vi "aggregation-lifetime-management.vi"(8 "error in (no error)":errorcluster) -> (0 "error out":errorcluster)   [LabVIEW 2013]
uses:
  src/SMO/SMO.lvclass
  <vilib>/addons/_JKI Toolkits/Caraya/classes/Test/Test.lvclass
  <vilib>/addons/_JKI Toolkits/Caraya/classes/Assert/Assert.lvclass
panel:
  # "<< Error 1556 illustrates a bug with version 1.1.7.31 \n\n(Essentially because B is destroyed by top-level before A is stopped, and A depends on B that no longer exists on stopping... this error should be handled by framework. Reverse the launching order to demonstrate bug is lifetime-related)"
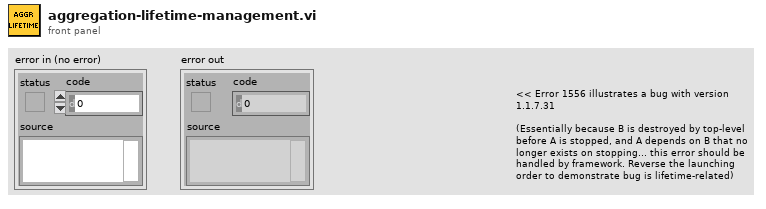
[diagram p1: front panel]
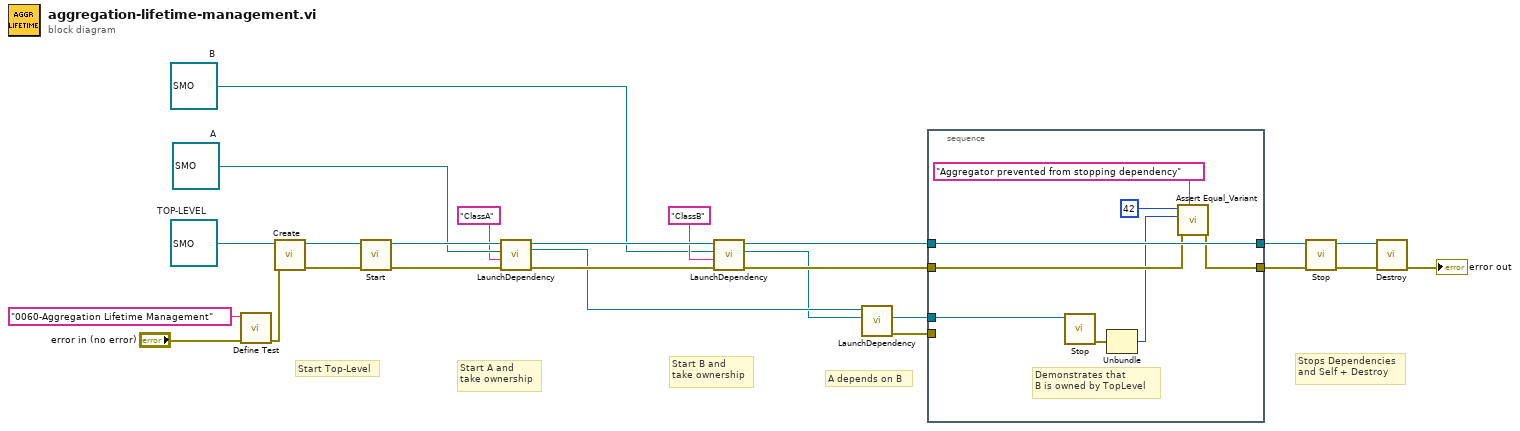
[diagram p0: block diagram]
diagram:
  w18 = refnum<class "SMO.lvclass"> refnum  # B
  w22 = refnum<class "SMO.lvclass"> refnum  # A
  w25 = refnum<class "SMO.lvclass"> refnum  # TOP-LEVEL
  # "Stops Dependencies\nand Self + Destroy"
  # "A depends on B"
  # "Start B and\ntake ownership"
  # "Start A and\ntake ownership"
  # "Start Top-Level"
  n1 = call <vilib>:"Define Test.vi"("error in (no error)"="error in (no error)", "Label (VI Title)"="0060-Aggregation Lifetime Management") -> ("error out"=w1:errorcluster)  [unwired: 9 in]
  n2 = call "Create.vi"("error in (no error)"=w1, "SMO"=w25) -> ("error out"=w16:errorcluster, "SMO out"=w24:refnum<class "SMO.lvclass">)  [unwired: 7 in, 1 out]
  n3 = call "Start.vi"("error in (no error)"=w16, "SMO"=w24) -> ("error out"=w17:errorcluster, "SMO out"=w23:refnum<class "SMO.lvclass">)  [unwired: 8 in]
  n4 = call "LaunchDependency.vi"("error in (no error)"=w17, "Dependency Name"="ClassA", "Dependency Type"=w22, "SMO in"=w23) -> ("error out"=w15:errorcluster, "Dependency Reference"=w6:refnum<class "SMO.lvclass">, "SMO out"=w20:refnum<class "SMO.lvclass">)  [unwired: 4 in, 1 out]
  n5 = call "LaunchDependency.vi"("error in (no error)"=w15, "Dependency Name"="ClassB", "Dependency Type"=w18, "SMO in"=w20) -> ("error out"=w12:errorcluster, "Dependency Reference"=w5:refnum<class "SMO.lvclass">, "SMO out"=w13:refnum<class "SMO.lvclass">)  [unwired: 4 in, 1 out]
  n6 = call "LaunchDependency.vi"("Dependency Type"=w5, "SMO in"=w6) -> ("error out"=w14:errorcluster, "Dependency Reference"=w11:refnum<class "SMO.lvclass">)  [unwired: 6 in, 2 out]
  n7 = stacked-sequence {
    tunnel: w14 -> [_]
    tunnel: w13 -> [w31]
    tunnel: w12 -> [w30]
    tunnel: w11 -> [w33]
    tunnel: [w31] -> w10
    tunnel: [w29] -> w9
    frame #0 {
      # "Demonstrates that\nB is owned by TopLevel"
      n8 = call "Stop.vi"("SMO"=w33) -> ("error out"=w32:errorcluster)  [unwired: 9 in, 1 out]
      n9 = Unbundle(w32) -> ("code"=w28:i32)  [unwired: 2 out]
      n10 = call <vilib>:"Assert Equal_Variant.vi"("Label"="Aggregator prevented from stopping dependency" ("Dependency Name"), "error in (no error)"=w30, "Y"=w28, "X"=42 ("y")) -> ("error out"=w29:errorcluster)  [unwired: 7 in]
    }
  }
  n11 = call "Stop.vi"("error in (no error)"=w9, "SMO"=w10) -> ("error out"=w7:errorcluster, "SMO out"=w8:refnum<class "SMO.lvclass">)  [unwired: 8 in]
  n12 = call "Destroy.vi"("error in (no error)"=w7, "SMO"=w8) -> ("error out"=→"error out":errorcluster)  [unwired: 9 in]
